vi "exmple1.vi"() -> ()   [LabVIEW 2017]
panel:
  out "Numeric":i32
  in  "stop":bool
  out "Waveform Graph":dbl[](graph)
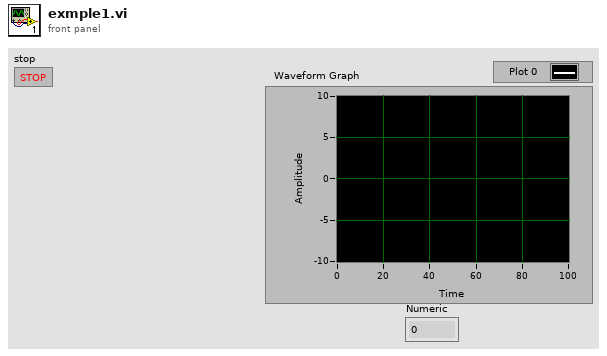
[diagram p1: front panel]
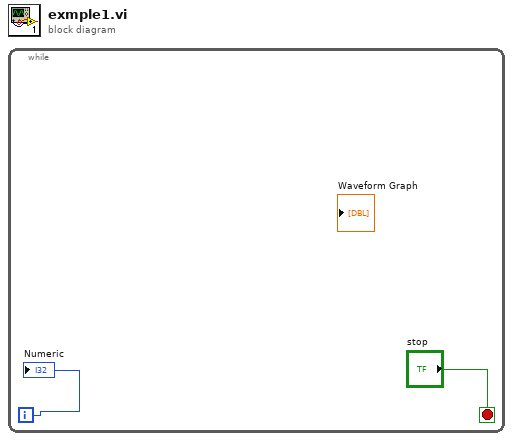
[diagram p0: block diagram]
diagram:
  n1 = while {
    i -> [w1]
    stop <- "stop" stop-if-true
    "Numeric" <- w1
  }
